vi "Create Virtual Instrument.vi"(8 "error in":errorcluster, 10 "Virtual Instrument Identifier":string) -> (0 "error out":errorcluster, 2 "IVirtual Instrument out":refnum<class "IVirtual Instrument.lvclass">)   [LabVIEW 2019, in "Instrument Manager.lvclass"]
uses:
  Instrument Manager.lvclass
  Instrument Manager.lvclass/Instrument Manager.ctl
  Interfaces/IUnmanaged/IUnmanaged.lvclass
  Config from JSON/Config from JSON.lvclass
  Interfaces/IVirtual Instrument/IVirtual Instrument.lvclass
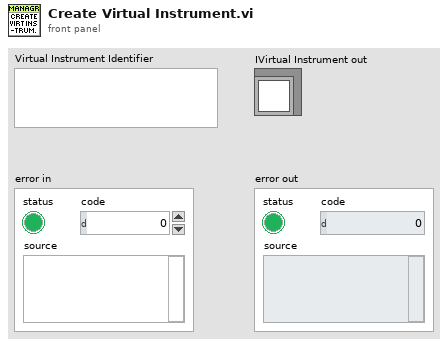
[diagram p1: front panel]
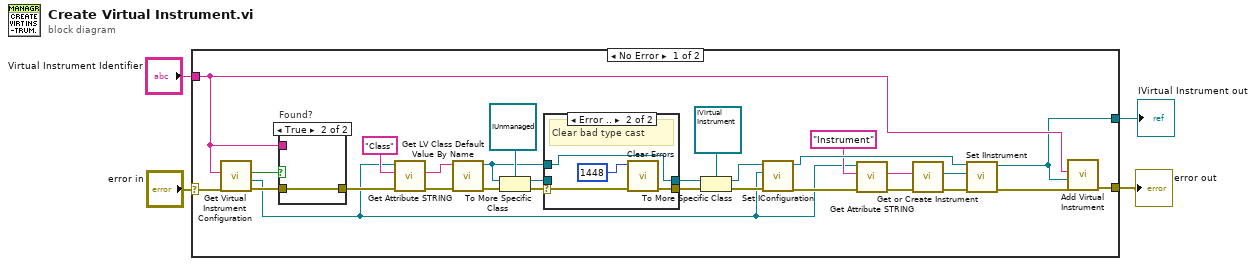
[diagram p0: block diagram]
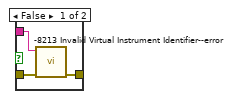
[diagram p2: hidden frame]
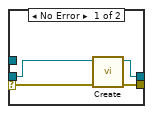
[diagram p3: hidden frame]
diagram:
  n1 = case shown="No Error" "error in" {
    selector: "error in" -> [w18 w46]
    tunnel: [w29 w46] -> w3
    tunnel: "Virtual Instrument Identifier" -> [w17 _]
    tunnel: [w8 _] -> w1
    frame No Error {
      n2 = call "Get Virtual Instrument Configuration.vi"("Error In"=w18, "Virtual Instrument Identifier"=w17) -> ("Error Out"=w27:errorcluster, "Virtual Instrument Configuration"=w9:refnum<class "Config from JSON.lvclass">, "Found"=w28:bool)  [unwired: 7 in]
      n3 = case "Found?" shown="True" w28 {
        tunnel: w27 -> [w36 w37]
        tunnel: [w35 w37] -> w26
        tunnel: w17 -> [w34 _]
        frame False {
          n4 = call "-8213 Invalid Virtual Instrument Identifier--error.vi"("error in"=w36, "Virtual Instrument Identifier"=w34) -> ("error out"=w35:errorcluster)  [unwired: 9 in]
        }
        frame True {
        }
      }
      n5 = call-dynamic "Get Attribute STRING.vi"("error in"=w26, "Attribute"="Class", "ConfigFromJSON in"=w9) -> ("error out"=w19:errorcluster, "Value"=w32:string)  [unwired: 6 in, 1 out]
      n6 = call <vilib>:"Get LV Class Default Value By Name.vi"("error in (no error)"=w19, "class name"=w32) -> ("error out"=w31:errorcluster, "object"=w16:refnum<class>)  [unwired: 8 in]
      n7 = To More Specific Class(target class=refnum<class "IUnmanaged.lvclass"> refnum ("IUnmanaged.lvclass"), reference=w16, error in=w31) -> (specific class reference=w22:refnum<class "IUnmanaged.lvclass">, error out=w25:errorcluster)
      n8 = case shown="Error .." w25 {
        selector: w25 -> [w41 w45]
        tunnel: [w40 w44] -> w23
        tunnel: w22 -> [w39 _]
        tunnel: [w38 w42] -> w21
        tunnel: w16 -> [_ w42]
        frame No Error {
          n9 = call-dynamic "Create.vi"("error in"=w41, "IUnmanaged in"=w39) -> ("error out"=w40:errorcluster, "IUnmanaged out"=w38:refnum<class "IUnmanaged.lvclass">)  [unwired: 8 in]
        }
        frame Error {
          # "Clear bad type cast"
          n10 = call <vilib>:"Clear Errors.vi"("error in (no error)"=w45, "specific error code to clear (0: all)"=1448) -> ("error out"=w44:errorcluster)  [unwired: 4 in, 1 out]
        }
      }
      n11 = To More Specific Class(target class=refnum<class "IVirtual Instrument.lvclass"> refnum ("IVirtual Instrument.lvclass"), reference=w21, error in=w23) -> (specific class reference=w24:refnum<class "IVirtual Instrument.lvclass">, error out=w15:errorcluster)
      n12 = call-dynamic "Set IConfiguration.vi"("error in"=w15, "IConfiguration"=w9, "IHasConfiguration in"=w24) -> ("error out"=w13:errorcluster, "IHasConfiguration out"=w14:refnum<class "IVirtual Instrument.lvclass">)  [unwired: 7 in]
      n13 = call-dynamic "Get Attribute STRING.vi"("error in"=w13, "Attribute"="Instrument", "ConfigFromJSON in"=w9) -> ("error out"=w11:errorcluster, "Value"=w10:string)  [unwired: 6 in, 1 out]
      n14 = call "Get or Create Instrument.vi"("Error In"=w11, "Instrument Identifier"=w10) -> ("Error Out"=w6:errorcluster, "IInstrument"=w7:refnum<class "IInstrument.lvclass">)  [unwired: 8 in]
      n15 = call-dynamic "Set IInstrument.vi"("error in"=w6, "IInstrument"=w7, "IVirtual Instrument in"=w14) -> ("error out"=w5:errorcluster, "IVirtual Instrument out"=w8:refnum<class "IVirtual Instrument.lvclass">)  [unwired: 7 in]
      n16 = call "Add Virtual Instrument.vi"("Error In"=w5, "IVirtual Instrument"=w8, "Instrument Identifier"=w17) -> ("Error Out"=w29:errorcluster)  [unwired: 8 in]
    }
    frame Error {
    }
  }
  "error out" <- w3
  "IVirtual Instrument out" <- w1
